vi "Set Int.vi"(8 "error in (no error)":errorcluster, 10 "Int":i32, 11 "IIntStatic (Named SEQ) in":refnum<class "IIntStatic (Named SEQ).lvclass">) -> (0 "error out":errorcluster, 3 "IIntStatic (Named SEQ) out":refnum<class "IIntStatic (Named SEQ).lvclass">)   [LabVIEW 2009, in "IIntStatic (Named SEQ).lvclass"]
uses:
  IIntStatic (Named SEQ).lvclass
  Numeric Test Object.lvclass
  Source/IUnknown Class/IUnknown.lvclass
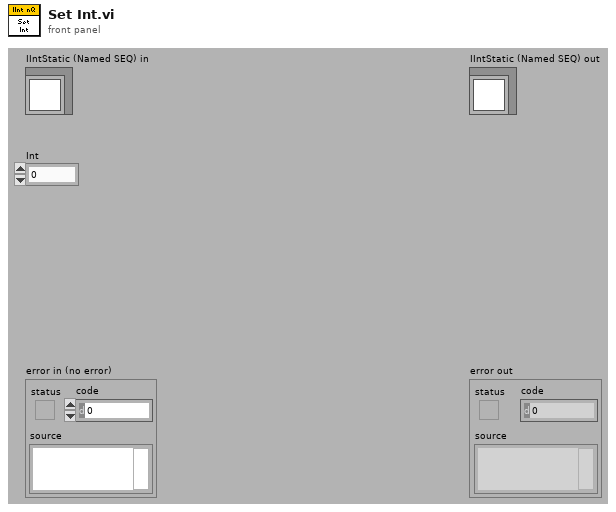
[diagram p1: front panel]
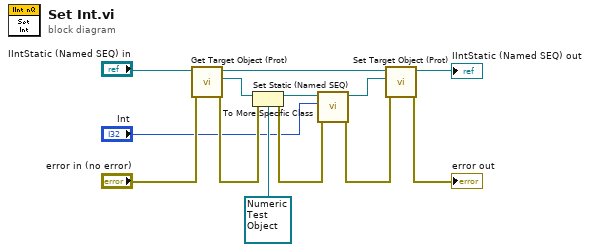
[diagram p0: block diagram]
diagram:
  n1 = call "Get Target Object (Prot).vi"("error in (no error)"="error in (no error)", "IUnknown in"="IIntStatic (Named SEQ) in") -> ("error out"=w12:errorcluster, "Target Object"=w13:refnum<class "Interfaceable.lvclass">, "IUnknown out"=w8:refnum<class "IIntStatic (Named SEQ).lvclass">)  [unwired: 7 in]
  n2 = To More Specific Class(target class=refnum<class "Numeric Test Object.lvclass"> refnum ("Numeric"), reference=w13, error in=w12) -> (specific class reference=w10:refnum<class "Numeric Test Object.lvclass">, error out=w9:errorcluster)
  n3 = call-dynamic "Set Static (Named SEQ).vi"("error in (no error)"=w9, "Int"="Int", "Numeric in"=w10) -> ("error out"=w6:errorcluster, "Numeric out"=w7:refnum<class "Numeric Test Object.lvclass">)  [unwired: 7 in]
  n4 = call "Set Target Object (Prot).vi"("error in (no error)"=w6, "Target Object"=w7, "IUnknown in"=w8) -> ("error out"=→"error out":errorcluster, "IUnknown out"=→"IIntStatic (Named SEQ) out":refnum<class "IIntStatic (Named SEQ).lvclass">)  [unwired: 7 in]
